vi "reg unreg for MacroGUI.vi"(7 "T for reg, F for unreg":bool, 8 "error in (no error)":errorcluster, 10 "event cluster":T1, 11 "Event Registration Refnum":refnum<event-registration>) -> (0 "error out":errorcluster, 3 "Event Registration Refnum Out":refnum<event-registration>)   [LabVIEW 2012]
doc: "SciScan 1.2 160622"
uses:
  <vilib>/Utility/VariantDataType/Type.ctl
  HFG/Custom Controls and Typedefs/HB Actionable Event.ctl
  <vilib>/Utility/miscctls.llb/LVRowAndColumnUnsignedTypeDef.ctl
  <vilib>/Utility/VariantDataType/VariantType.lvlib
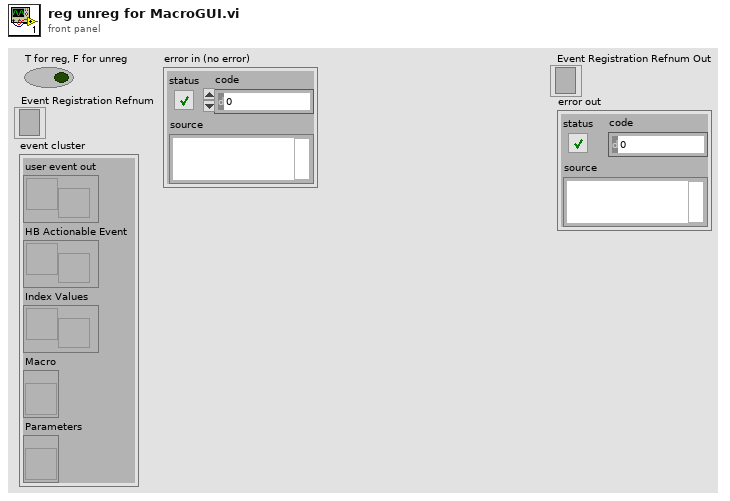
[diagram p1: front panel]
types:
  T1 = cluster{"user event out":refnum<user-event>, "HB Actionable Event":refnum<user-event>, "Index Values":refnum<user-event>, "Macro":refnum<vi>, "Parameters":refnum<vi>}
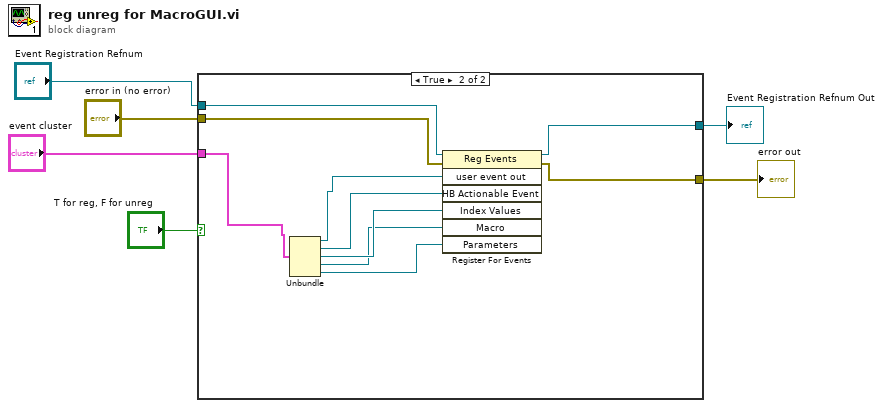
[diagram p0: block diagram]
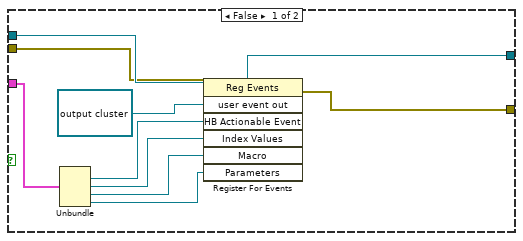
[diagram p2: hidden frame]
diagram:
  n1 = case shown="True" "T for reg, F for unreg" {
    tunnel: "event cluster" -> [w13 w26]
    tunnel: "Event Registration Refnum" -> [w15 w20]
    tunnel: [w14 w19] -> w3
    tunnel: "error in (no error)" -> [w8 w17]
    tunnel: [w7 w18] -> w1
    frame False {
      n2 = Unbundle(w13) -> ("HB Actionable Event"=w12:refnum<user-event>, "Index Values"=w11:refnum<user-event>, "Macro"=w10:refnum<vi>, "Parameters"=w9:refnum<vi>)  [unwired: 1 out]
      n3 = register-events(reference=w15, error in=w8, refnum<user-event> refnum ("event source"), w12, w11, w10, w9) -> (reference out=w14:refnum<event-registration>, error out=w7:errorcluster)
    }
    frame True {
      n4 = Unbundle(w26) -> ("user event out"=w25:refnum<user-event>, "HB Actionable Event"=w24:refnum<user-event>, "Index Values"=w23:refnum<user-event>, "Macro"=w22:refnum<vi>, "Parameters"=w21:refnum<vi>)
      n5 = register-events(reference=w20, error in=w17, w25, w24, w23, w22, w21) -> (reference out=w19:refnum<event-registration>, error out=w18:errorcluster)
    }
  }
  "Event Registration Refnum Out" <- w3
  "error out" <- w1
